vi "HE_reg.vi"(0 "HE_reg in":refnum<class "HE_reg.lvclass">, 1 "Y":T2={"Y_HSw"=1, "Y_HSetState"=enum."auto", "Y_ASetState"=enum."auto", "Y_DSetState"=enum."auto"}, 2 "Z":cluster{"Z_State":T6, "ZM_State":T7}={"Z_State"=enum."alarm", "ZM_State"=enum."initialization"}, 3 "XB24 (F)":bool, 5 "SP":dbl caption="setpoint" step=0.01 format="%.2f", 7 "PV":dbl step=0.01 format="%.2f", 9 "PV_State":T1, 11 "error in (no error)":errorcluster, 12 "Y_H":dbl step=1.0, 13 "controls Y":cluster{"Y_L":dbl, "Y_A":dbl, "Y_D":dbl} {"Y_D" format="%#_13g"; "Y_A" format="%#_13g"; "Y_L" format="%.2f"}) -> (4 "HE_reg out":refnum<class "HE_reg.lvclass">, 6 "Y_State":T4={"Y_Source"=enum."local disabled", "Y_SetState"=enum."auto", "SP_Set"=0.0, "SP"=0.0, "PV"=0.0, "Y_Set"=0.0, "Y"=0.0, "Y_State"={"code"=0, "visible"=FALSE, "color"=0}, "YB"=FALSE} {"Y_Set" format="%.2f"; "SP" step=0.01 format="%.2f"; "Y" format="%.2f"; "PV" step=0.01 format="%.2f"; "SP_Set" step=0.01 format="%.2f"}, 8 "Y":dbl format="%.2f", 10 "YB":bool, 15 "error out":errorcluster)   [LabVIEW 2019, in "Heating.lvlib" / "HE_reg.lvclass"]
uses:
  HE_reg.lvclass
  D:/my_projects/projects/Algorithms/Labview/19/Reg/PID/PID_OL_AM/PID_OL_AM.lvclass
  ctl/Z_State.ctl
  ctl/ZM_State.ctl
  ctl/Y_short.ctl
  ctl/Y_source.ctl
  ctl/Y_state.ctl
  Inputs/Ctl/Parameter State short.ctl
  ctl/Y_control.ctl
  Reg/ctl/SpLim_State.ctl
  HE_reg.lvclass/HE_reg.ctl
  Reg/PID/PID SP Limiter/PID SP Limiter.lvclass/PID SP Limiter.ctl
  Reg/PID/PID Output Rate Limiter/PID Output Rate Limiter.lvclass/PID Output Rate Limiter.ctl
  Reg/PID/PID Timing Estimation/PID Timing Estimation.lvclass/PID Timing Estimation.ctl
  Reg/PID/PID_OL_AM/PID_OL_AM.lvclass/PID_OL_AM.ctl
  Transform/Impulsator.lvclass/Impulsator.ctl
  Reg/PID/PID Output Rate Limiter/PID Output Rate Limiter.vi
  Reg/PID/PID Output Rate Limiter/Write output rate.vi
  Reg/PID/PID Timing Estimation/PID Timing Estimation.vi
  Reg/PID/PID Output Rate Limiter/Read output.vi
  Reg/PID/PID SP Limiter/PID SP Limiter.lvclass
  D:/my_projects/projects/Algorithms/Labview/19/Reg/PID/PID Output Rate Limiter/PID Output Rate Limiter.lvclass
  Reg/PID/PID Output Rate Limiter/PID Output Rate Limiter.lvclass
  D:/my_projects/projects/Algorithms/Labview/19/Reg/PID/PID Timing Estimation/PID Timing Estimation.lvclass
  Reg/PID/PID_OL_AM/PID_OL_AM.lvclass
  Heating.lvlib
  Reg/control.lvlib
  Transform/Impulsator.lvclass
  Inputs/Inputs.lvlib
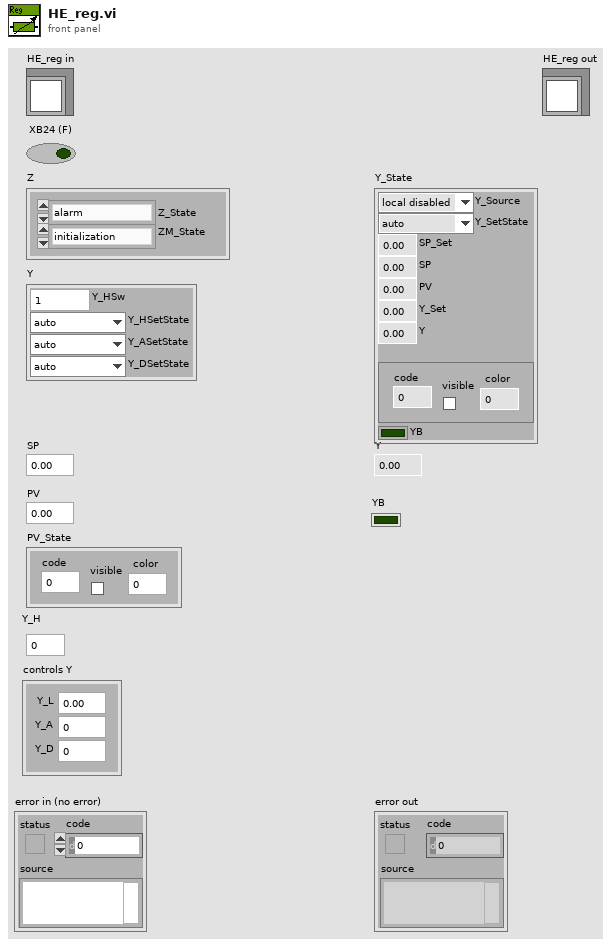
[diagram p1: front panel]
types:
  T1 = typedef "Inputs.lvlib/Parameter State short.ctl" = cluster{"code":i32, "visible":bool, "color":u32}
  T2 = typedef "Heating.lvlib/Y_control.ctl" = cluster{"Y_HSw":u8, "Y_HSetState":T3, "Y_ASetState":T3, "Y_DSetState":T3}
  T3 = typedef "Heating.lvlib/Y_state.ctl" = enum8{"initialize", "alarm", "min", "stop", "hand", "auto", "max"}
  T4 = typedef "Heating.lvlib/Y_short.ctl" = cluster{"Y_Source":T5, "Y_SetState":T3, "SP_Set":dbl, "SP":dbl, "PV":dbl, "Y_Set":dbl, "Y":dbl, "Y_State":T1, "YB":bool}
  T5 = typedef "Heating.lvlib/Y_source.ctl" = enum8{"initialize", "local disabled", "local hand", "hand", "auto", "dist"}
  T6 = typedef "Heating.lvlib/Z_State.ctl" = enum8{"initialization", "alarm", "disabled", "not ready", "stop ready", "reserv", "switched off", "reserv2", "switched on", "check", "on min", "decrease out", "on", "increase out", "on max"}
  T7 = typedef "Heating.lvlib/ZM_State.ctl" = enum8{"initialization", "stop", "start_cmd", "contactor_on_cmd", "heating", "on", "stop_cmd", "power_down", "contactor_off_cmd", "cooling", "restart_delay"}
  T8 = typedef "control.lvlib/SpLim_State.ctl" = enum8{"initialization", "stop", "decrease", "increase"}
  T9 = enum8{"alarm", "min", "stop", "hand", "auto", "max"}
  T10 = cluster{"Y_Source":T5, "Y_SetState":T3, "SP":dbl, "output":dbl, "PV":dbl, "pid output":dbl, "rate lim output":dbl, "PV_State":T1, "YB":bool}
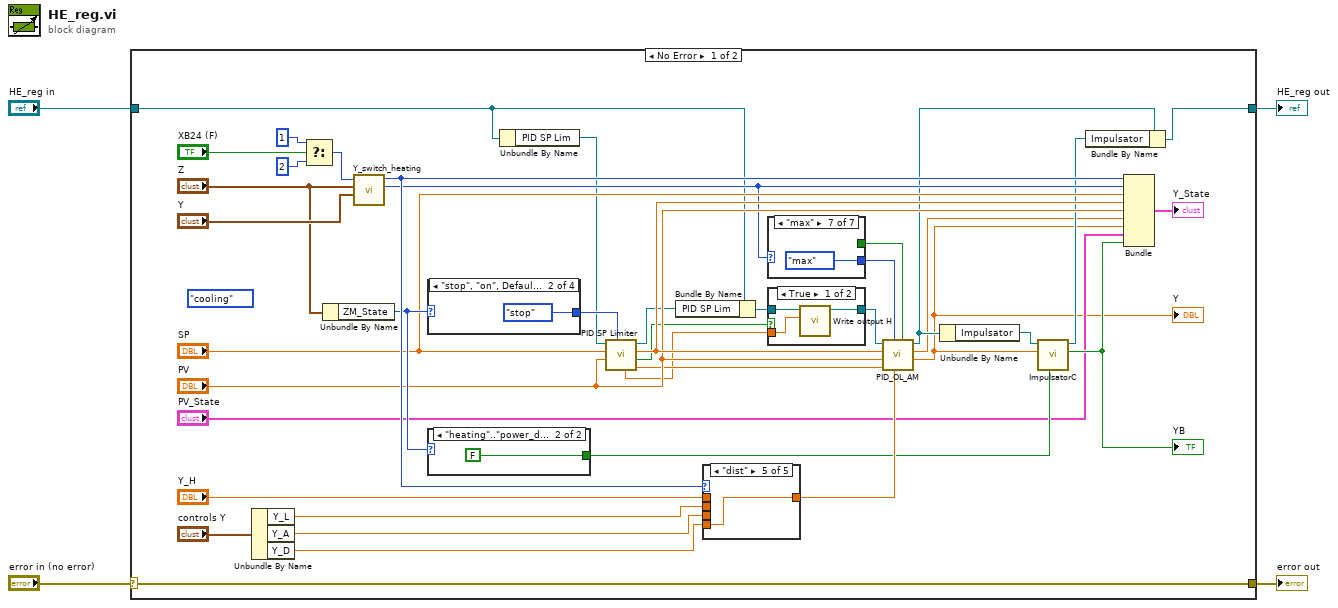
[diagram p0: block diagram]
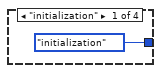
[diagram p2: hidden frame]
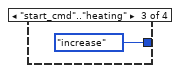
[diagram p3: hidden frame]
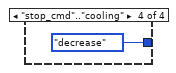
[diagram p4: hidden frame]
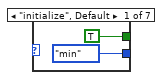
[diagram p6: hidden frame]
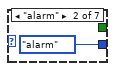
[diagram p7: hidden frame]
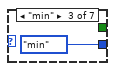
[diagram p8: hidden frame]
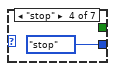
[diagram p9: hidden frame]
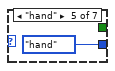
[diagram p10: hidden frame]
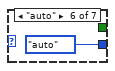
[diagram p11: hidden frame]
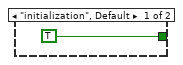
[diagram p12: hidden frame]
diagram:
  n1 = case shown="No Error" "error in (no error)" {
    selector: "error in (no error)" -> [w44 w69]
    tunnel: [w44 w69] -> w3
    tunnel: [w16 w68] -> w1
    tunnel: "HE_reg in" -> [w14 w68]
    frame No Error {
      (unwired) ZM_State."cooling" ("ZM_State")
      n2 = Unbundle By Name("controls Y") -> ("Y_L"=w41:dbl, "Y_A"=w42:dbl, "Y_D"=w40:dbl)
      n3 = Select(t=u8 1, s="XB24 (F)", f=u8 2 ("Y_HSw")) -> (s? t:f=w36:u8)
      n4 = Unbundle By Name("Z") -> ("ZM_State"=w29:T7)
      n5 = call "Y_switch_heating.vi"("Y"="Y", "Z"="Z", "Y_LSw (2-auto)"=w36) -> ("Y_SetState"=w24:T3, "Y_Source"=w34:T5)  [unwired: 7 in]
      n6 = case shown="\"stop\", \"on\", Default" w29 {
        tunnel: [SpLim_State."initialization" ("SpLim_State") SpLim_State."stop" ("SpLim_State") SpLim_State."increase" ("SpLim_State") SpLim_State."decrease" ("SpLim_State")] -> w30
        frame "initialization" {
        }
        frame "stop", "on", Default {
        }
        frame "start_cmd".."heating" {
        }
        frame "stop_cmd".."cooling" {
        }
      }
      n7 = case shown="\"heating\"..\"power_down\"" w29 {
        tunnel: [TRUE FALSE] -> w15
        frame "initialization", Default {
        }
        frame "heating".."power_down" {
        }
      }
      n8 = Unbundle By Name(w14) -> ("PID SP Lim"=w20:refnum<class "PID SP Limiter.lvclass">)
      n9 = call "PID SP Limiter.vi"("SpLim_State"=w30, "PV"="PV", "SP"="SP", "PID SP Limiter in"=w20) -> ("dt (s) out"=w19:dbl, "SpLim_State changed"=w13:bool, "output"=w27:dbl, "PID SP Limiter out"=w21:refnum<class "PID SP Limiter.lvclass">, "pid_out_H"=w10:dbl)  [unwired: 3 in]
      n10 = Bundle By Name(cluster=w14, "PID SP Lim"=w21) -> (w12:refnum<class "HE_reg.lvclass">)
      n11 = case shown="\"dist\"" w34 {
        tunnel: "Y_H" -> [_ _ w65 _ _]
        tunnel: w41 -> [w63 w64 _ _ _]
        tunnel: w40 -> [_ _ _ _ w67]
        tunnel: [w63 w64 w65 w66 w67] -> w25
        tunnel: w42 -> [_ _ _ w66 _]
        frame "local disabled", Default {
        }
        frame "local hand" {
        }
        frame "hand" {
        }
        frame "auto" {
        }
        frame "dist" {
        }
      }
      n12 = case shown="\"max\"" w24 {
        tunnel: [T9."min" ("X1(SetState)") T9."alarm" ("X1(SetState)") T9."min" ("X1(SetState)") T9."stop" ("X1(SetState)") T9."hand" ("X1(SetState)") T9."auto" ("X1(SetState)") T9."max" ("X1(SetState)")] -> w23
        tunnel: [TRUE _ _ _ _ _ _] -> w22
        frame "initialize", Default {
        }
        frame "alarm" {
        }
        frame "min" {
        }
        frame "stop" {
        }
        frame "hand" {
        }
        frame "auto" {
        }
        frame "max" {
        }
      }
      n13 = case shown="True" w13 {
        tunnel: w12 -> [w51 w52]
        tunnel: [w50 w52] -> w11
        tunnel: w10 -> [w49 _]
        frame True {
          n14 = call "Write output H.vi"("output H"=w49, "PID_OL_AM in"=w51) -> ("PID_OL_AM out"=w50:refnum<class "HE_reg.lvclass">)  [unwired: 9 in]
        }
        frame False {
        }
      }
      n15 = call "PID_OL_AM.vi"("reinitialize? (F)"=w22, "manual control"=w25, "X1(SetState)"=w23, "dt (s) in"=w19, "process variable"="PV", "setpoint"=w27, "PID in"=w11) -> ("rate lim output"=w6:dbl, "pid output"=w5:dbl, "PID out"=w9:refnum<class "HE_reg.lvclass">)  [unwired: 1 in, 1 out]
      "Y" <- w6
      n16 = Unbundle By Name(w9) -> ("Impulsator"=w18:refnum<class "Impulsator.lvclass">)
      n17 = call "ImpulsatorC.vi"("Initialise"=w15, "PV"=w6, "Impulsator in"=w18) -> ("YB"=w8:bool, "Impulsator out"=w17:refnum<class "Impulsator.lvclass">)  [unwired: 7 in]
      "YB" <- w8
      n18 = Bundle By Name(cluster=w9, "Impulsator"=w17) -> (w16:refnum<class "HE_reg.lvclass">)
      n19 = Bundle("Y_Source"=w34, "Y_SetState"=w24, "SP"="SP", "output"=w27, "PV"="PV", "pid output"=w5, "rate lim output"=w6, "PV_State"="PV_State", "YB"=w8) -> (→"Y_State":T10)  [unwired: 1 in]
    }
    frame Error {
    }
  }
  "error out" <- w3
  "HE_reg out" <- w1
